vi "Send Software Trigger.vi"(8 "error in (no error)":errorcluster, 9 "Trigger Mode (1: Analog)":i32(ring)=1 items=["Digitize", "Analog"], 10 "Buffer Name (\"\")":string, 11 "VISA resource name":refnum<visa-resource-name>) -> (0 "error out":errorcluster, 3 "VISA resource name out":refnum<visa-resource-name>)   [LabVIEW 2015, in "Keithley DMM6500 DAQ6500 Series.lvlib"]
doc: "Sends a trigger to the instrument. After each call to the <b>Initiate</b> VI, send a trigger by calling this VI. When triggers are complete, call the <b>Fetch (Multiple)</b> VI. \n\n<B>Note:</B> Use this VI only with other low-level VIs. The high-level VIs automatically incorporate this functionality. \n\nTypically, you call this VI only in a sequence of calls to other low-level instrument driver VIs. The sequence performs one operation. You use the low-level VIs to optimize one or more aspects of interaction with the instrument."
uses:
  <instrlib>/Keithley DMM6500 DAQ6500 Series/Keithley DMM6500 DAQ6500 Series.lvlib
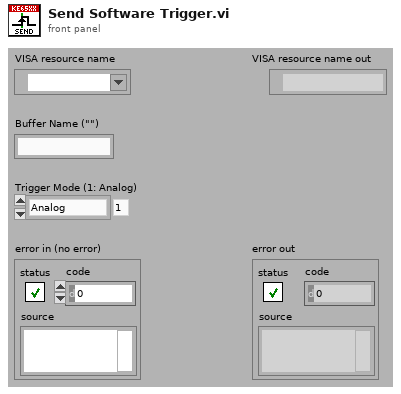
[diagram p1: front panel]
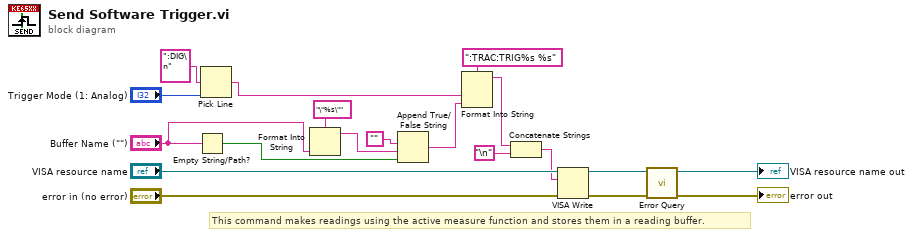
[diagram p0: block diagram]
diagram:
  # "This command makes readings using the active measure function and stores them in a reading buffer."
  n1 = Empty String/Path?(string/path="Buffer Name (\"\")") -> (empty?=w5:bool)
  n2 = Pick Line(multi-line string=":DIG\n", line index="Trigger Mode (1: Analog)") -> (output string=w7:string)  [unwired: 1 in]
  n3 = Format Into String(format string="\"%s\"", "Buffer Name (\"\")") -> (resulting string=w10:string)  [unwired: 2 in, 1 out]
  n4 = Append True/False String(1:w5, 2:w10, 3:"") -> (0:w12:string)  [unwired: 1 in]
  n5 = Format Into String(format string=":TRAC:TRIG%s %s", w7, w12) -> (resulting string=w15:string)  [unwired: 2 in, 1 out]
  n6 = Concatenate Strings(w15, "\n") -> (w16:string)
  n7 = VISA Write(VISA resource name="VISA resource name", write buffer=w16, error in (no error)="error in (no error)") -> (VISA resource name out=w4:refnum<visa-resource-name>, error out=w3:errorcluster)  [unwired: 1 out]
  n8 = call <instrlib>:"Error Query.vi"("error in (no error)"=w3, "VISA resource name"=w4) -> ("error out"=→"error out":errorcluster, "VISA resource name out"=→"VISA resource name out":refnum<visa-resource-name>)  [unwired: 6 in, 2 out]
